vi "myFreqSymm.vi"(8 "基频":u32=50, 10 "响应测试选项":u8(ring)=2 items=["仅测量信号", "单相扫频", "三相同步系扫频", "三相正负序扫频"], 11 "Freqs in":i32[](array[numeric])=[10, 14, 19, 27, 37, 51, 71, 99, 140, 190, 260, 360, 510, 700, 970, 1400, 1900, 2600, 3600, 5000]) -> (3 "Freqs out":i32[](array[numeric]))   [LabVIEW 2024]
doc: "当待测正负序耦合时：\n1）在原扫频点集基础上扩充密度。\n2）在正频点后面补充一个负轴频点组，用于负序注入的情况。\n当待测同步系耦合时：\n1）从频点组中去掉基波，这是因为dsp端（大概）不能注入直流。"
uses:
  fd1eec49-f234-40ac-bef1-b501cdfe1280.vi
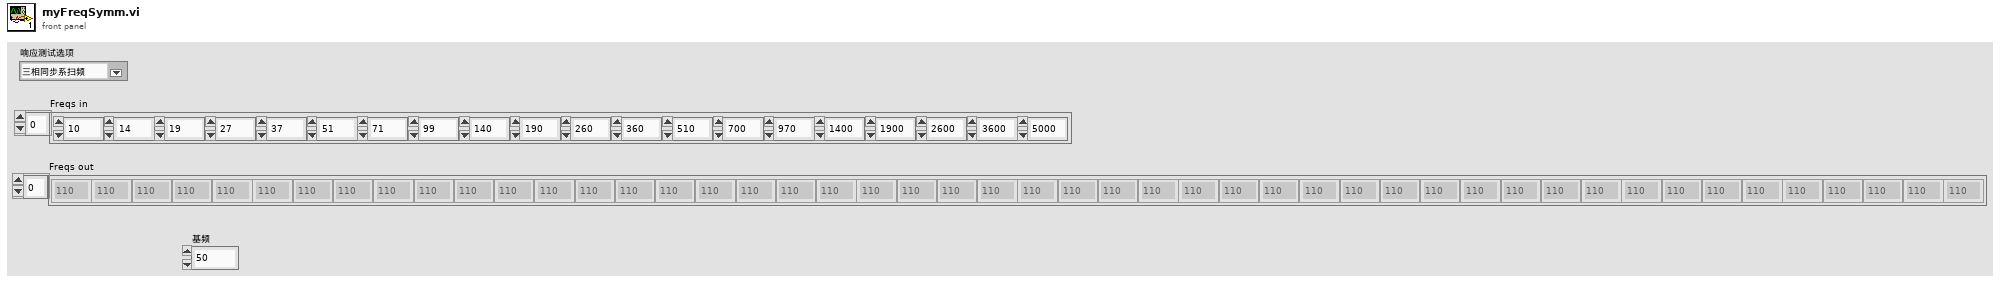
[diagram p1: front panel]
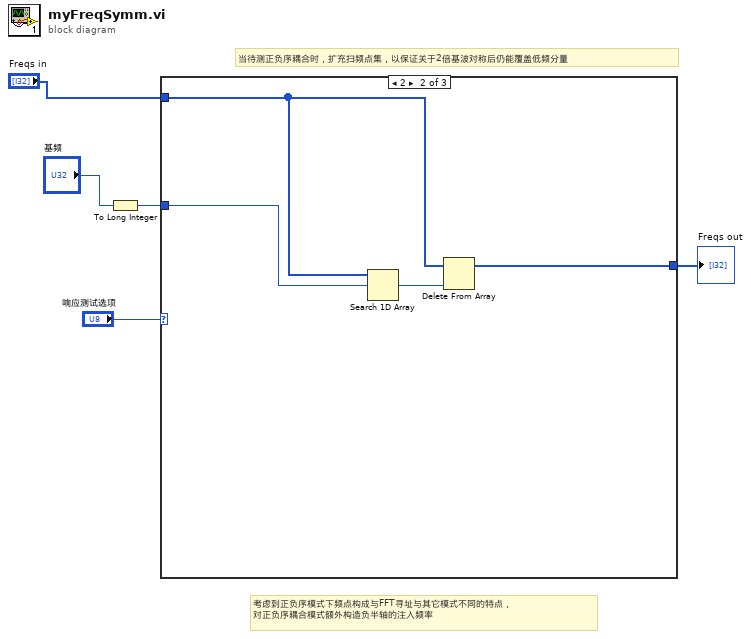
[diagram p0: block diagram]
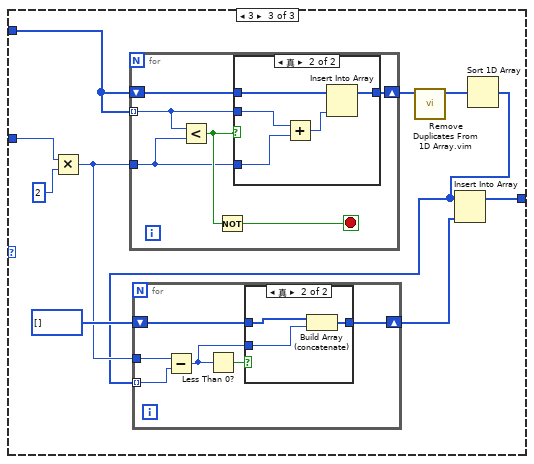
[diagram p3: hidden frame]
diagram:
  # "考虑到正负序模式下频点构成与FFT寻址与其它模式不同的特点，\n对正负序耦合模式额外构造负半轴的注入频率"
  # "当待测正负序耦合时，扩充扫频点集，以保证关于2倍基波对称后仍能覆盖低频分量"
  n1 = To Long Integer(number="基频") -> (32bit integer=w4:i32)
  n2 = case shown="2" "响应测试选项" {
    tunnel: "Freqs in" -> [w6 w9 w18]
    tunnel: [w6 w8 w12] -> w5
    tunnel: w4 -> [_ w7 w15]
    frame 0, Default {
    }
    frame 2 {
      n3 = Search 1D Array(1D array=w9, element=w7) -> (index of element=w10:i32)  [unwired: 1 in]
      n4 = Delete From Array(array=w9, index=w10) -> (array with subset deleted=w8:i32[])  [unwired: 1 in, 1 out]
    }
    frame 3 {
      n5 = Multiply(x=w15, y=2) -> (x*y=w14:i32)
      n6 = for {
        tunnel: w18 -> [w32] mode=indexing
        shift-right: [w33] -> w20
        shift-left: w18 -> [w34]
        tunnel: w14 -> [w31]
        stop <- w36 stop-if-true
        n7 = Less?(x=w32, y=w31) -> (x < y?=w35:bool)
        n8 = Not(x=w35) -> (.not. x?=w36:bool)
        n9 = case shown="真" w35 {
          tunnel: w34 -> [w37 w42]
          tunnel: [w37 w41] -> w33
          tunnel: w32 -> [_ w40]
          tunnel: w31 -> [_ w38]
          frame False {
          }
          frame True {
            n10 = Add(x=w40, y=w38) -> (x+y=w39:i32)
            n11 = Insert Into Array(array=w42, new element=w39) -> (w41:i32[])  [unwired: 1 in]
          }
        }
      }
      n12 = call "Remove Duplicates From 1D Array.vim"("array"=w20) -> ("array with duplicates removed"=w19:i32[])  [unwired: 10 in]
      n13 = Sort 1D Array(array=w19) -> (sorted array=w11:i32[])
      n14 = for {
        tunnel: w11 -> [w23] mode=indexing
        shift-right: [w25] -> w13
        shift-left: i32[] [] -> [w26]
        tunnel: w14 -> [w24]
        n15 = Subtract(x=w24, y=w23) -> (x-y=w21:i32)
        n16 = Less Than 0?(x=w21) -> (x < 0?=w22:bool)
        n17 = case shown="真" w22 {
          tunnel: w26 -> [w27 w30]
          tunnel: [w27 w29] -> w25
          tunnel: w21 -> [_ w28]
          frame False {
          }
          frame True {
            n18 = Build Array (concatenate)(w30, w28) -> (w29:i32[])
          }
        }
      }
      n19 = Insert Into Array(array=w11, new element=w13) -> (w12:i32[])  [unwired: 1 in]
    }
  }
  "Freqs out" <- w5
